vi "Init_Test.vi"(8 "error in (no error)":errorcluster caption="entrée d'erreur (pas d'erreur)", 11 "Flash_Jlink en entrée":refnum<class "P2265_SwitchOff_Test.lvclass">) -> (0 "error out":errorcluster caption="sortie d'erreur", 3 "Flash_Jlink en sortie":refnum<class "P2265_SwitchOff_Test.lvclass">)   [LabVIEW 2020, in "Library Test.lvlib" / "P2265_SwitchOff_Test.lvclass"]
uses:
  P2265_SwitchOff_Test.lvclass
  C:/Users/ngarcin/OneDrive - Altyor/Standard TB/Class/Test/Test (Default)/Test (Default).lvclass
  Commun VI/TypeDef/Commande Test/Commande Type Test.ctl
  Commun VI/TypeDef/Commande Test/Commande Value Type.ctl
  Test_Wtih_Instr/Test_With_Inst.lvclass
  P2265_SwitchOff_Test.lvclass/P2265_SwitchOff_Test.ctl
  Commun VI/Library Commun.lvlib
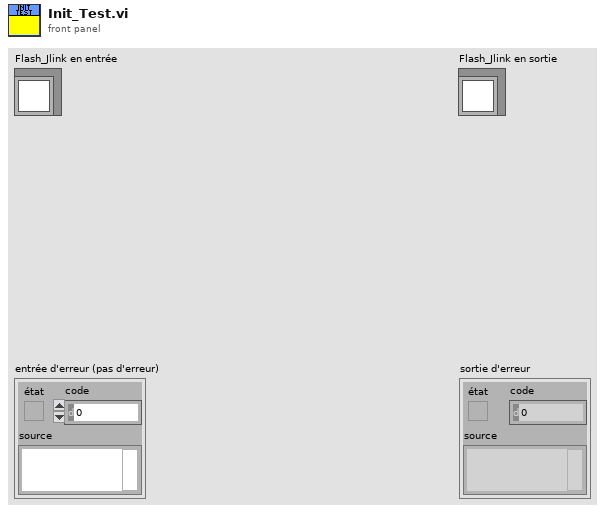
[diagram p1: front panel]
types:
  T1 = typedef "Library Commun.lvlib/Commande Value Type.ctl" = enum16{"None", "String", "Number", "Timestamp", "Boolean", "Array"}
  T2 = typedef "Library Commun.lvlib/Commande Type Test.ctl" = enum16{"Function", "Test", "Calculation"}
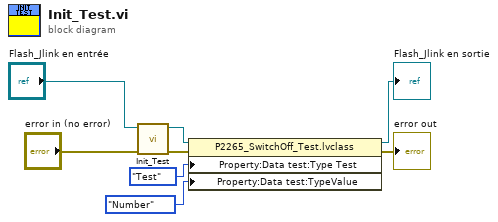
[diagram p0: block diagram]
diagram:
  n1 = call-parent "Init_Test.vi"("error in (no error)"="error in (no error)", "Test_With_Inst en entrée"="Flash_Jlink en entrée") -> ("error out"=w3:errorcluster, "Test_With_Inst en sortie"=w5:refnum<class "P2265_SwitchOff_Test.lvclass">)  [unwired: 8 in]
  n2 = property class="P2265_SwitchOff_Test.lvclass"(reference=w5, error in=w3, "Property:Data test:Type Test"=Commande_Type_Test."Test" ("Type Test"), "Property:Data test:TypeValue"=Commande_Value_Type."Number" ("TypeValue")) -> (reference out=→"Flash_Jlink en sortie":refnum<class "P2265_SwitchOff_Test.lvclass">, error out=→"error out":errorcluster)
